vi "dfd_Set Unit Option.vi"(8 "error in (no error)":errorcluster, 9 "fs [Hz]":dbl=1000.0 format="%.2f", 10 "unit option":u16(ring) items=["Samples", "Seconds"], 11 "freq responses":cluster{"f0":dbl, "df":dbl, "values":dbl[]}[](array[cluster]) {"df" format="%.2f"; "f0" format="%.2f"; "values" format="%.2f"}) -> (0 "error out":errorcluster, 3 "freq responses out":cluster{"f0":dbl, "df":dbl, "values":dbl[]}[](array[cluster]))   [LabVIEW 2017, in "NI_DigFilterLicensed.lvlib"]
uses:
  <vilib>/addons/Digital Filter Design/NI_DigFilterLicensed.lvlib
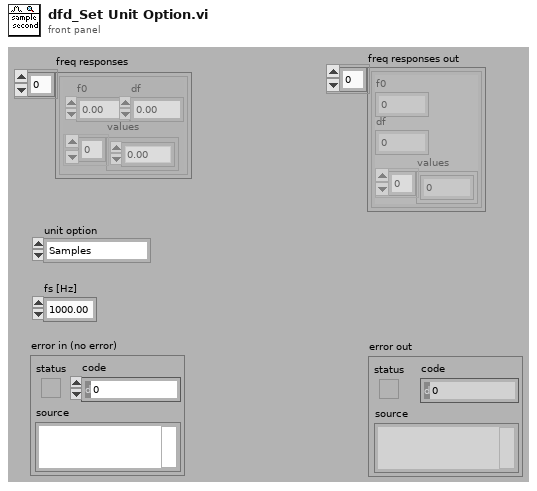
[diagram p1: front panel]
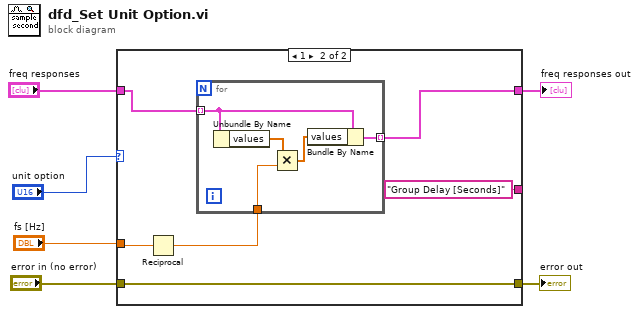
[diagram p0: block diagram]
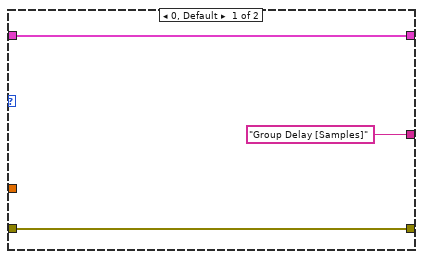
[diagram p2: hidden frame]
diagram:
  n1 = case shown="1" "unit option" {
    tunnel: "freq responses" -> [w9 w14]
    tunnel: [w9 w13] -> w3
    tunnel: "fs [Hz]" -> [_ w15]
    tunnel: [w8 w11] -> w2
    tunnel: "error in (no error)" -> [w8 w11]
    tunnel: ["Group Delay [Samples]" "Group Delay [Seconds]"] -> _
    frame 0, Default {
    }
    frame 1 {
      n2 = Reciprocal(x=w15) -> (1/x=w12:dbl)
      n3 = for {
        tunnel: w14 -> [w19] mode=indexing
        tunnel: [w20] -> w13 mode=indexing
        tunnel: w12 -> [w17]
        n4 = Unbundle By Name(w19) -> ("values"=w18:dbl[])
        n5 = Multiply(x=w18, y=w17) -> (x*y=w16:dbl[])
        n6 = Bundle By Name(cluster=w19, "values"=w16) -> (w20:cluster{"f0":dbl, "df":dbl, "values":dbl[]})
      }
    }
  }
  "freq responses out" <- w3
  "error out" <- w2
